vi "Constants.vi"() -> ()   [LabVIEW 2019, in "RefMem DMA Shared.lvlib"]
doc: "Use this Global VI to access the GUIDs assigned to the page resources of the Custom Device."
uses:
  RefMem DMA Shared.lvlib
panel:
  in  "Tab Control":enum32{"GUIDS", "Constants", "Properties"}(tab)
  out "Decimation Channel GUID":string="8433dcab-dea3-4110-97cf-311a1b3fd76d"
  out "Status Section GUID":string="782d9ef4-3de5-4e4c-bb43-83b54ca0e2a2"
  out "Del Prot Chan GUID":string="e91a84f3-78c7-400a-8e17-8c81a2c16c94"
  in  "Data Folder":string="8c1ebf08-4571-4c85-9af4-c2761dbfdef8"
  in  "Data Channel":string="1ad56b5b-8f49-4d01-a2b2-7e5717d92d0c"
  in  "RefMem DMA":string="0e1a756e-1a6e-416d-924d-af2409f2f6d8"
  out "CSV File Path":string="CSV File Path"
  in  "Compiled.Settings":string="Compiled.Settings"
  out "Block Address":string="Block Address"
  out "CPU":string="CPU"
  out "Type":string="Type"
  out "VISA Name":string="VISA Name"
  out "Relative Address in Block":string="Relative Address in Block"
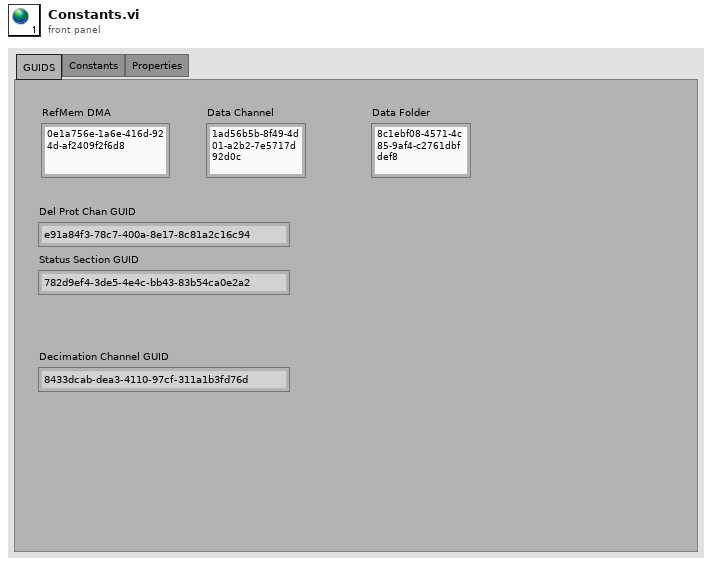
[diagram p1: front panel]
diagram:
